vi "CCD_CheckError.vi"(0 "CCD GPIB Address":i16=1 min=1 max=1, 5 "Mode":T1(ring)=enum."Check CCD Command Error", 7 "milliseconds to wait":u32, 11 "error in":errorcluster) -> (1 "Poll Byte":i16, 2 "Poll Status":bool[](array[boolean]), 4 "SRQ":bool, 6 "CCD Error?":bool, 8 "Error (0=No Error)":i16=-1, 12 "Status#2":bool[](array[boolean]), 13 "Returned String":string, 14 "Bytes Read":u8[](array[numeric]), 15 "error out":errorcluster)   [LabVIEW 2019]
doc: "(1) Poll CCD\n(2) Check CCD Command Error\n(3) Check CCD SRQ Status, if true, porform a serial poll.\n\nTwo status arrays are returned: \"Poll Status\" is always meaningful and \"Status #2\" is the GPIB status after operation #2, i.e., Read in Mode (2) and SPoll in Mode (3)."
uses:
  Globals and TypeDefs/Error Categories.ctt
panel:
  out "hex values Read":string[](array[string])
  out "SetupTime (ms)":u32=3
  # "Status Byte Explanations:\n[0]: Dev.Clear State  \n[1]: Dev.Trig.State    \n[2]: Listener Active   \n[3]: Talker Active      \n[4]: Attn. Asserted    \n[5]: CIC                      \n[6]: Remote State       \n[7]: Lockout State      \n[8]: Oper.Complete\n[9]:   ---\n[10]: ---\n[11]: ---\n[12]: SRQ det.whl CIC\n[13]: EOI or EOS det.\n[14]: Timeout\n[15]: Error detected"
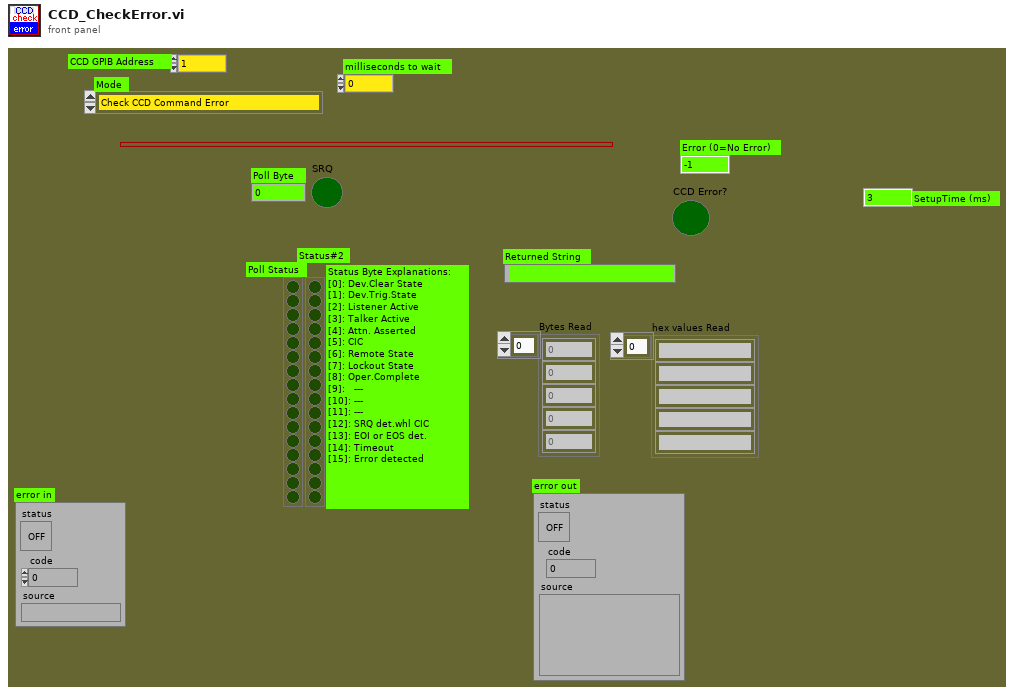
[diagram p1: front panel]
types:
  T1 = enum16{"Poll CCD GPIB Status", "Check CCD Command Error", "CheckSRQ-Poll"}
  T2 = enum8{"Initialization Error", "Command Error", "Parameter Error", "Overflow Error", "Time-out Error", "Misc Error", "User cancel"}
  T3 = typedef "Error Categories.ctt" = enum8{"General", "CCD-256x1024", "CCD-1340x400", "InGaAs PDA", "McPherson 2075", "Magnetic Field", "Temperature Control", "Other"}
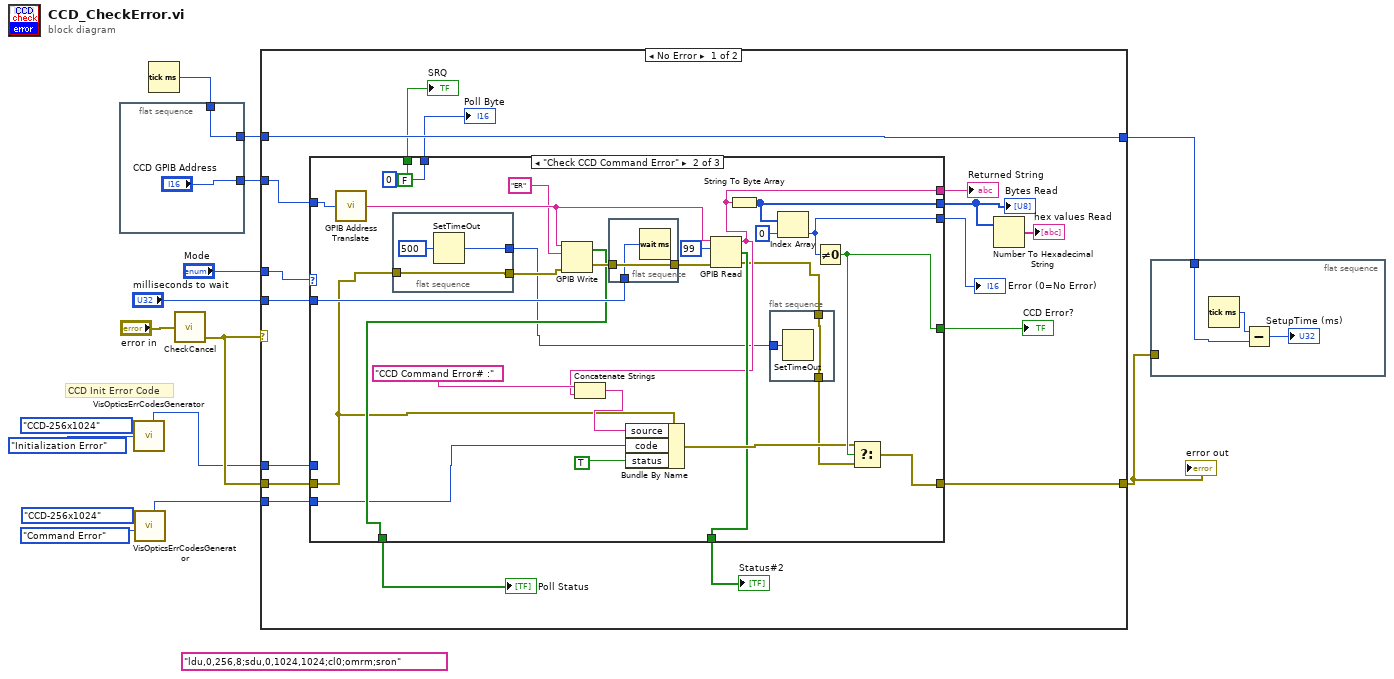
[diagram p0: block diagram]
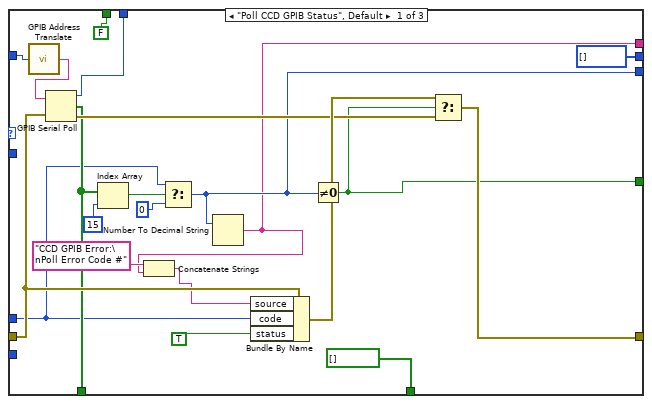
[diagram p2: hidden frame]
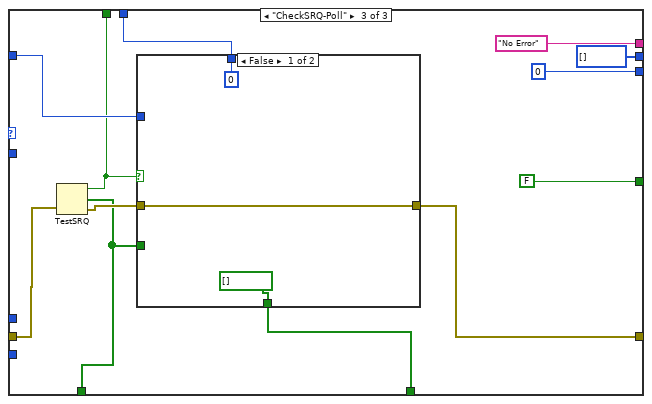
[diagram p3: hidden frame]
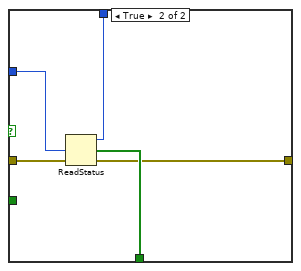
[diagram p4: hidden frame]
diagram:
  (unwired) "ldu,0,256,8;sdu,0,1024,1024;cl0;omrm;sron"
  # "CCD Init Error Code"
  n1 = flat-sequence {
    tunnel: ["CCD GPIB Address"] -> w12
    tunnel: w13 -> [w16]
    tunnel: [w16] -> w9
    frame #0 {
    }
  }
  n2 = call "VisOpticsErrCodesGenerator.vi"("NHMFL Visible Optics Error Type"=T2."Initialization Error", "NHMFL Visible Optics Error Categories"=Error_Categories.ctt."CCD-256x1024") -> ("User-defined Error Code"=w6:i32)  [unwired: 1 in, 5 out]
  n3 = call "VisOpticsErrCodesGenerator.vi"("NHMFL Visible Optics Error Type"=T2."Command Error", "NHMFL Visible Optics Error Categories"=Error_Categories.ctt."CCD-256x1024") -> ("User-defined Error Code"=w1:i32)  [unwired: 1 in, 5 out]
  n4 = Tick Count (ms)() -> (millisecond timer value=w13:u32)
  n5 = call "CheckCancel.vi"("error in (no error)"="error in") -> ("error out"=w14:errorcluster)  [unwired: 1 in, 1 out]
  n6 = case shown="No Error" w14 {
    tunnel: w14 -> [w34 w111]
    tunnel: [w33 w111] -> w10
    tunnel: w12 -> [w32 _]
    tunnel: w6 -> [w31 _]
    tunnel: "Mode" -> [w30 _]
    tunnel: [w29 w110] -> w8
    tunnel: w9 -> [w29 w110]
    tunnel: "milliseconds to wait" -> [w26 _]
    tunnel: w1 -> [w18 _]
    frame No Error {
      n7 = case shown="\"Check CCD Command Error\"" w30 {
        tunnel: w34 -> [w51 w62 w95]
        tunnel: w32 -> [w39 w73 w98]
        tunnel: [w50 w75 w94] -> w33
        tunnel: w31 -> [w35 _ _]
        tunnel: [w45 w64 0 ("t")] -> w28
        tunnel: [w44 w77 FALSE] -> w27
        tunnel: w26 -> [_ w74 _]
        tunnel: [w43 w63 "No Error" ("data")] -> w20
        tunnel: [w42 i16 0 ("serial poll response") w96] -> w25
        tunnel: [w41 w68 w91] -> w24
        tunnel: [FALSE ("SRQ") FALSE ("SRQ") w93] -> w23
        tunnel: [bool[] [] ("status") w67 w92] -> w22
        tunnel: [u8[] [] ("unsigned byte array") w66 u8[] [] ("unsigned byte array")] -> w19
        tunnel: w18 -> [_ w57 _]
        frame "Poll CCD GPIB Status", Default {
          n8 = call "GPIB Address Translate.vi"("GPIB Address"=w39) -> ("GPIB Address String"=w38:string)
          n9 = GPIB Serial Poll(0:w38, 1:w51) -> (2:w42:i16, 3:w41:bool[], 4:w46:errorcluster)
          n10 = Index Array(array=w41, index=15) -> (element=w54:bool)
          n11 = Select(t=w35, s=w54, f=i16 0) -> (s? t:f=w45:i32)
          n12 = Number To Decimal String(number=w45) -> (decimal integer string=w43:string)  [unwired: 1 in]
          n13 = Concatenate Strings("CCD GPIB Error:\nPoll Error Code #" ("string"), w43) -> (w49:string)
          n14 = Bundle By Name(cluster=w51, "source"=w49, "code"=w35, "status"=TRUE) -> (w47:errorcluster)
          n15 = Not Equal To 0?(x=w45) -> (x != 0?=w44:bool)
          n16 = Select(t=w47, s=w44, f=w46) -> (s? t:f=w50:errorcluster)
        }
        frame "Check CCD Command Error" {
          n17 = call "GPIB Address Translate.vi"("GPIB Address"=w73) -> ("GPIB Address String"=w70:string)
          n18 = flat-sequence {
            tunnel: w62 -> [w87]
            tunnel: [w87] -> w61
            tunnel: [w85] -> w58
            frame #0 {
              n19 = SetTimeOut(1:500 ("new timeout (10000)")) -> (0:w85:i32)
            }
          }
          n20 = GPIB Write(0:w70, 1:"ER" ("data string"), 3:w61) -> (5:w68:bool[], 6:w82:errorcluster)  [unwired: 2 in]
          n21 = flat-sequence {
            tunnel: w82 -> [w89]
            tunnel: [w89] -> w81
            tunnel: w74 -> [w88]
            frame #0 {
              n22 = Wait (ms)(milliseconds to wait=w88) -> ()  [unwired: 1 out]
            }
          }
          n23 = GPIB Read(0:w70, 1:99 ("byte count"), 3:w81) -> (5:w63:string, 6:w67:bool[], 7:w60:errorcluster)  [unwired: 2 in]
          n24 = Concatenate Strings("CCD Command Error# :" ("string"), w63) -> (w80:string)
          n25 = Bundle By Name(cluster=w62, "source"=w80, "code"=w57, "status"=TRUE) -> (w76:errorcluster)
          n26 = String To Byte Array(string=w63) -> (unsigned byte array=w66:u8[])
          n27 = flat-sequence {
            tunnel: w60 -> [w84]
            tunnel: [w84] -> w59
            tunnel: w58 -> [w83]
            frame #0 {
              n28 = SetTimeOut(1:w83) -> ()  [unwired: 1 out]
            }
          }
          n29 = Index Array(array=w66, index=0) -> (element=w64:u8)
          n30 = Not Equal To 0?(x=w64) -> (x != 0?=w77:bool)
          n31 = Select(t=w76, s=w77, f=w59) -> (s? t:f=w75:errorcluster)
        }
        frame "CheckSRQ-Poll" {
          n32 = TestSRQ(1:w95) -> (2:w93:bool, 3:w91:bool[], 4:w97:errorcluster)  [unwired: 1 in]
          n33 = case shown="False" w93 {
            tunnel: w98 -> [_ w109]
            tunnel: w97 -> [w104 w108]
            tunnel: [bool[] [] ("status") w107] -> w92
            tunnel: [i16 0 ("serial poll response") w106] -> w96
            tunnel: [w104 w105] -> w94
            tunnel: w91 -> [_ _]
            frame False {
            }
            frame True {
              n34 = ReadStatus(3:w108, 4:w109) -> (0:w105:errorcluster, 1:w107:bool[], 2:w106:i16)  [unwired: 1 in]
            }
          }
        }
      }
      "CCD Error?" <- w27
      "Returned String" <- w20
      "SRQ" <- w23
      "Bytes Read" <- w19
      "Error (0=No Error)" <- w28
      "Poll Byte" <- w25
      "Poll Status" <- w24
      "Status#2" <- w22
      n35 = Number To Hexadecimal String(2:w19) -> (0:→"hex values Read":string[])  [unwired: 1 in]
    }
    frame Error {
    }
  }
  "error out" <- w10
  n36 = flat-sequence {
    tunnel: w10 -> [_]
    tunnel: w8 -> [w112]
    frame #0 {
      n37 = Tick Count (ms)() -> (millisecond timer value=w113:u32)
      n38 = Subtract(x=w113, y=w112) -> (x-y=→"SetupTime (ms)":u32)
    }
  }
